vi "Lorentz_2D.vi"(3 "output control":T1, 4 "data":T2, 5 "X":dbl[](array[numeric]), 6 "a":dbl[](array[numeric])) -> (0 "error out":errorcluster, 1 "f'(X,a)":dbl[][](array[numeric]), 2 "f(X,a)":dbl[](array[numeric]))   [LabVIEW 2014]
doc: "This VI conforms the the template needed for use with the nonlinear fit function. This computes a 2D Lorentzian where the array 'a' has elements as follows:\n\nAmplitude\nX Position\nY Position\nFWHM\nOffset"
uses:
  <vilib>/gmath/NumericalOptimization/objective function data.ctl
  <vilib>/gmath/NumericalOptimization/LM_output select.ctl
  <vilib>/gmath/NI_Gmath.lvlib
panel:
  # "X Array can be all zeros, it just sets the image size (square)"
  # "Amp\nXo\nYo\nWidth\nOffset"
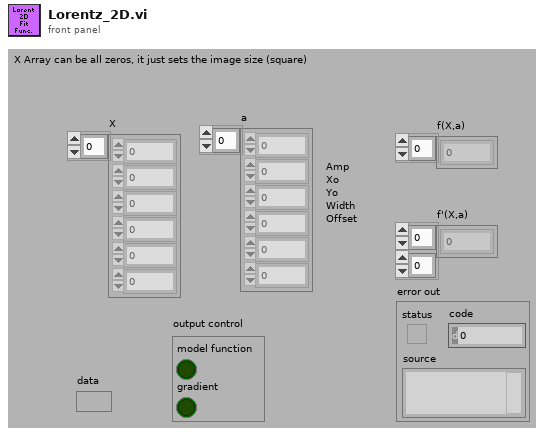
[diagram p1: front panel]
types:
  T1 = typedef "NI_Gmath.lvlib/LM_output select.ctl" = cluster{"model function":bool, "gradient":bool}
  T2 = typedef "NI_Gmath.lvlib/objective function data.ctl" = variant
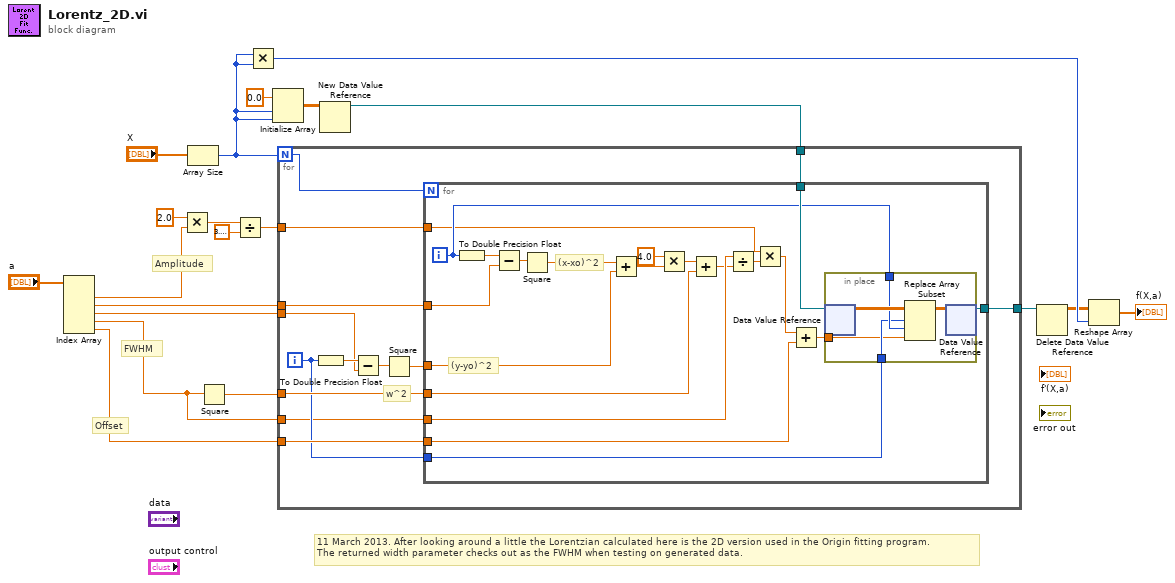
[diagram p0: block diagram]
diagram:
  # "Offset"
  # "FWHM"
  # "Amplitude"
  # "11 March 2013. After looking around a little the Lorentzian calculated here is the 2D version used in the Origin fitting program.\nThe returned width parameter checks out as the FWHM when testing on generated data."
  n1 = Index Array(array="a") -> (element #1=w5:dbl, element #2=w18:dbl, element #3=w17:dbl, element #4=w2:dbl, element #5=w12:dbl)  [unwired: 5 in]
  n2 = Multiply(x=2.0, y=w5) -> (x*y=w3:dbl)
  n3 = Array Size(array="X") -> (size(s)=w8:i32)
  n4 = Square(x=w2) -> (x^2=w9:dbl)
  n5 = Divide(x=w3, y=3.141592653589793) -> (x/y=w10:dbl)
  n6 = Multiply(x=w8, y=w8) -> (x*y=w6:i32)
  n7 = Initialize Array(0.0 ("element"), w8, w8) -> (w15:dbl[][])
  n8 = New Data Value Reference(data value=w15) -> (data value reference=w14:refnum<data-value>)  [unwired: 1 in, 1 out]
  n9 = for {
    N: w8 -> [w33]
    tunnel: w10 -> [w32]
    tunnel: w18 -> [w31]
    tunnel: w17 -> [w28]
    tunnel: w12 -> [w30]
    tunnel: w9 -> [w25]
    tunnel: w14 -> [w24]
    tunnel: [w22] -> w13
    tunnel: w2 -> [w21]
    i -> [w23]
    # "w^2"
    n10 = To Double Precision Float(number=w23) -> (double precision float=w29:dbl)
    n11 = Subtract(x=w29, y=w28) -> (x-y=w27:dbl)
    n12 = Square(x=w27) -> (x^2=w26:dbl)
    n13 = for {
      N: w33 -> [_]
      tunnel: w32 -> [w37]
      tunnel: w31 -> [w52]
      tunnel: w30 -> [w35]
      tunnel: w26 -> [w45]
      tunnel: w25 -> [w44]
      tunnel: w24 -> [w50]
      tunnel: w23 -> [w48]
      tunnel: [w47] -> w22
      tunnel: w21 -> [w40]
      i -> [w49]
      # "(y-yo)^2"
      # "(x-xo)^2"
      n14 = To Double Precision Float(number=w49) -> (double precision float=w53:dbl)
      n15 = Subtract(x=w53, y=w52) -> (x-y=w51:dbl)
      n16 = Square(x=w51) -> (x^2=w46:dbl)
      n17 = Add(x=w46, y=w45) -> (x+y=w43:dbl)
      n18 = Multiply(x=4.0, y=w43) -> (x*y=w41:dbl)
      n19 = Add(x=w41, y=w44) -> (x+y=w39:dbl)
      n20 = Divide(x=w40, y=w39) -> (x/y=w38:dbl)
      n21 = Multiply(x=w37, y=w38) -> (x*y=w36:dbl)
      n22 = Add(x=w36, y=w35) -> (x+y=w34:dbl)
      n23 = in-place {
        in-place-border: w49 -> [w56]
        in-place-border: w48 -> [w55]
        in-place-border: w34 -> [w54]
        n24 = in-place-dvr #1(w50) -> (w58:dbl[][])  [unwired: 1 out]
        n25 = Replace Array Subset(array=w58, new element=w54, index (row)=w55, index (col)=w56) -> (w57:dbl[][])
        n26 = in-place-dvr #1(w57) -> (w47:refnum<data-value>)  [unwired: 1 out]
      }
    }
  }
  n27 = Delete Data Value Reference(data value reference=w13) -> (data value=w1:dbl[][])  [unwired: 1 in, 1 out]
  n28 = Reshape Array(w1, w6) -> (→"f(X,a)":dbl[])
